vi "SMCP1_CMD_INIT_ZERO.vi"(8 "Error In":errorcluster) -> (0 "Error Out":errorcluster, 3 "SMCP1_CMD_INIT_ZERO":i32)   [LabVIEW 2016, in "OSB_uMp_library.lvlib"]
doc: "Constant used as an argument to pass to ump_cmd function that represents an instruction to perform a calibration routine."
uses:
  OSB_uMp_library.lvlib
panel:
  # "By Stuart Box at OxSyBio Ltd, 2017\n\nThis software is provided WITHOUT ANY WARRANTY; without even the implied warranty of MERCHANTABILITY or FITNESS FOR A PARTICULAR PURPOSE.\n\ninfo@oxsybio.com\n\nOxSyBio Ltd, The Walbrook Building, 25 Walbrook, London, EC4N 8AF"
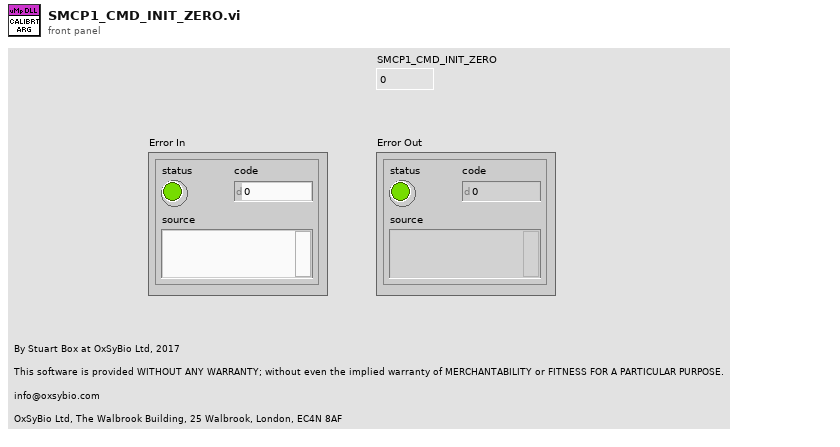
[diagram p1: front panel]
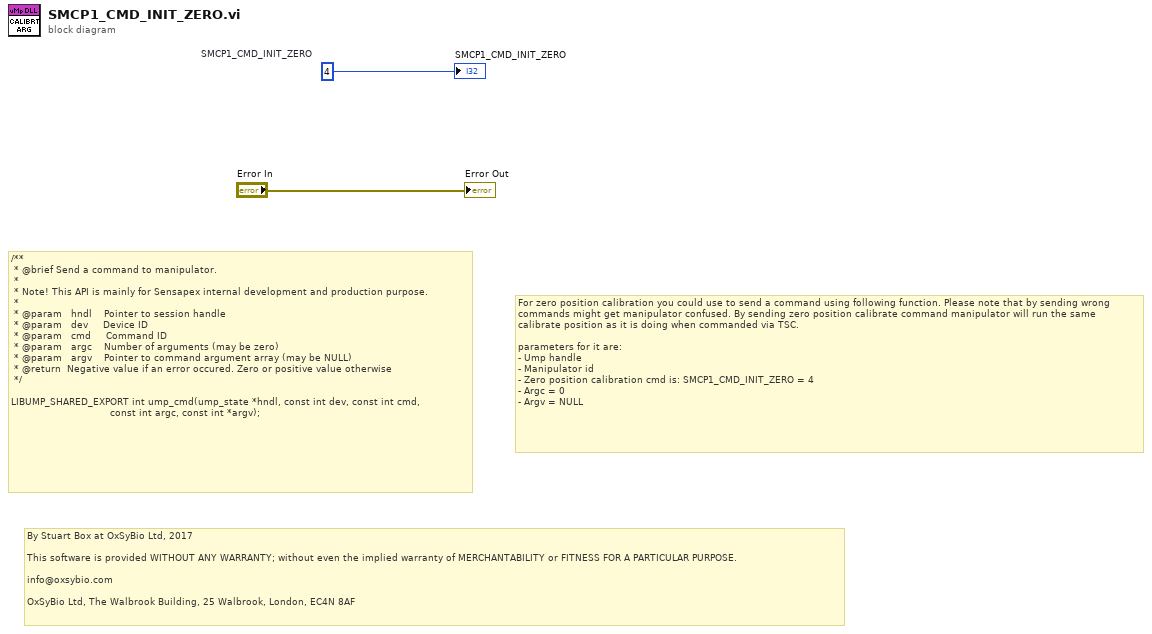
[diagram p0: block diagram]
diagram:
  w1 = 4  # SMCP1_CMD_INIT_ZERO
  # "By Stuart Box at OxSyBio Ltd, 2017\n\nThis software is provided WITHOUT ANY WARRANTY; without even the implied warranty of MERCHANTABILITY or FITNESS FOR A PARTICULAR PURPOSE.\n\ninfo@oxsybio.com\n\nOxSyBio Ltd, The Walbrook Building, 25 Walbrook, London, EC4N 8AF"
  # "For zero position calibration you could use to send a command using following function. Please note that by sending wrong commands might get manipulator confused. By sending zero position calibrate command manipulator will run the same calibrate position as it is doing when commanded via TSC.\n\nparameters for it are:\n-\tUmp handle\n-\tManipulator id\n-\tZero position calibration cmd is: SMCP1_CMD_INIT_ZERO = 4\n-\tArgc = 0\n-\tArgv = NULL"
  # "/**\n * @brief Send a command to manipulator.\n *\n * Note! This API is mainly for Sensapex internal development and production purpose.\n *\n * @param   hndl    Pointer to session handle\n * @param   dev     Device ID\n * @param   cmd     Command ID\n * @param   argc    Number of arguments (may be zero)\n * @param   argv    Pointer to command argument array (may be NULL)\n * @return  Negative value if an error occured. Zero or positive value otherwise\n */\n\nLIBUMP_SHARED_EXPORT int ump_cmd(ump_state *hndl, const int dev, const int cmd,\n                                 const int argc, const int *argv);"
  "Error Out" <- "Error In"
  "SMCP1_CMD_INIT_ZERO" <- w1
